vi "Get Type.vi"(8 "error in (no error)":errorcluster, 11 "Metal Case in":refnum<class "Metal Case.lvclass">) -> (0 "error out":errorcluster, 2 "Item Type":T1, 3 "Metal Case out":refnum<class "Metal Case.lvclass">)   [LabVIEW 2020, in "Metal Case.lvclass"]
uses:
  Metal Case.lvclass
  Item/Item Type.ctl
  Item/Item.lvclass
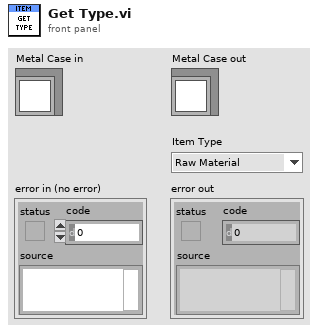
[diagram p1: front panel]
types:
  T1 = typedef "Item.lvclass/Item Type.ctl" = enum16{"Raw Material", "Component", "Module", "Product"}
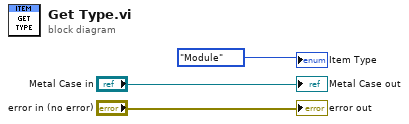
[diagram p0: block diagram]
diagram:
  "error out" <- "error in (no error)"
  "Metal Case out" <- "Metal Case in"
  "Item Type" <- Item_Type."Module" ("Item Type")
